vi "Controls Disable.vi"(10 "Controls in":refnum<vi>[](array[refnum])) -> ()   [LabVIEW 2025, in "_Shared.lvlib"]
uses:
  _Shared.lvlib
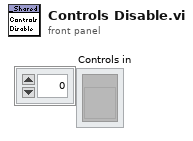
[diagram p1: front panel]
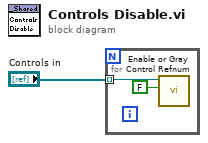
[diagram p0: block diagram]
diagram:
  n1 = for {
    tunnel: "Controls in" -> [w2] mode=indexing
    n2 = call <vilib>:"Enable or Gray Control Refnum.vi"("enable?"=FALSE, "Control in"=w2) -> ()  [unwired: 8 in, 2 out]
  }
